vi "Write Image Prefix.vi"(8 "error in (no error)":errorcluster, 10 "Prefix":string, 11 "HIJ IMAQdx Camera Viewer in":refnum<class "HIJ Vision Camera App.lvclass">) -> (0 "error out":errorcluster, 3 "HIJ IMAQdx Camera Viewer out":refnum<class "HIJ Vision Camera App.lvclass">)   [LabVIEW 2020, in "HIJ Vision Camera App.lvlib" / "HIJ Vision Camera App.lvclass"]
uses:
  HIJ Vision Camera App.lvclass
  HIJ Vision Camera App.lvclass/HIJ Vision Camera App.ctl
  HIJ Vision Application/HIJ Vision Application/HIJ Vision Application.lvclass
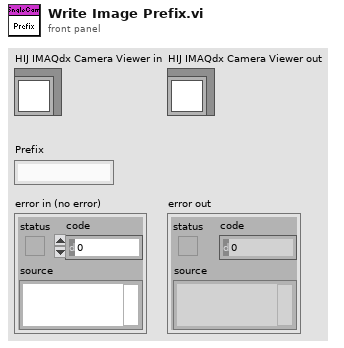
[diagram p1: front panel]
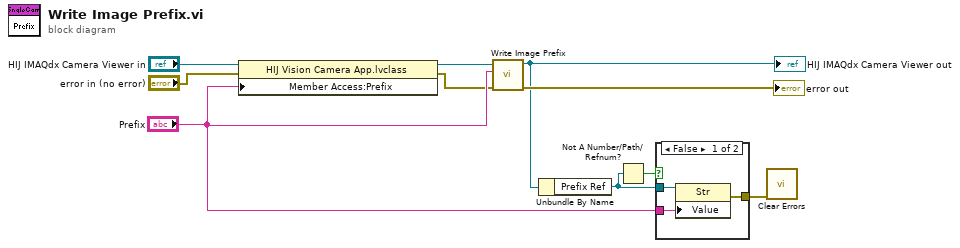
[diagram p0: block diagram]
diagram:
  n1 = property class="HIJ Vision Camera App.lvclass"(reference="HIJ IMAQdx Camera Viewer in", error in="error in (no error)", "Member Access:Prefix"="Prefix") -> (reference out=w4:refnum<class "HIJ Vision Camera App.lvclass">, error out=w1:errorcluster)
  n2 = call-parent "Write Image Prefix.vi"("error in (no error)"=w1, "Prefix"="Prefix", "HIJ Vision Application in"=w4) -> ("error out"=→"error out":errorcluster, "HIJ Vision Application out"=w7:refnum<class "HIJ Vision Camera App.lvclass">)  [unwired: 7 in]
  "HIJ IMAQdx Camera Viewer out" <- w7
  n3 = Unbundle By Name(w7) -> ("Prefix Ref"=w5:refnum<vi>)
  n4 = Not A Number/Path/Refnum?(number/path/refnum=w5) -> (NaN/Path/Refnum?=w6:bool)
  n5 = case shown="False" w6 {
    tunnel: w5 -> [w13 _]
    tunnel: "Prefix" -> [w12 _]
    tunnel: [w11 _] -> w9
    frame False {
      n6 = property class="Str"(reference=w13, "Value"=w12) -> (error out=w11:errorcluster)  [unwired: 1 in, 1 out]
    }
    frame True {
    }
  }
  n7 = call <vilib>:"Clear Errors.vi"("error in (no error)"=w9) -> ()  [unwired: 5 in, 2 out]
